vi "Read Cubes.vi"(8 "error in (no error)":errorcluster, 11 "Cubes in":refnum<class "Cubes.lvclass">) -> (0 "error out":errorcluster, 2 "Cubes":refnum<class "Cube.lvclass">[](array[class]), 3 "Cubes out":refnum<class "Cubes.lvclass">)   [LabVIEW 2019, in "22.lvlib" / "Cubes.lvclass"]
uses:
  Cubes.lvclass
  Cube/Cube.lvclass
  Cubes.lvclass/Cubes.ctl
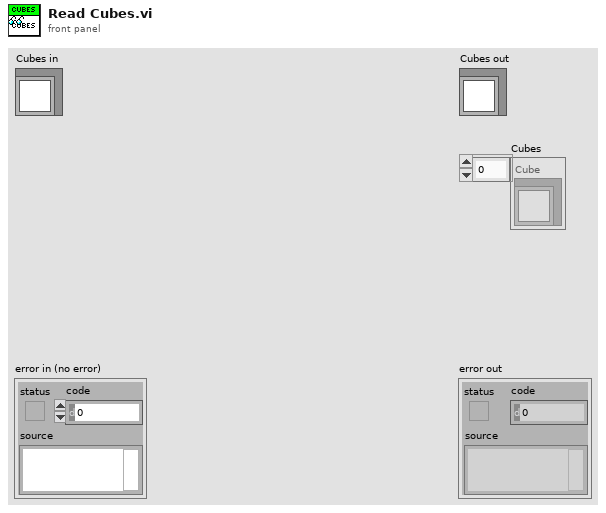
[diagram p1: front panel]
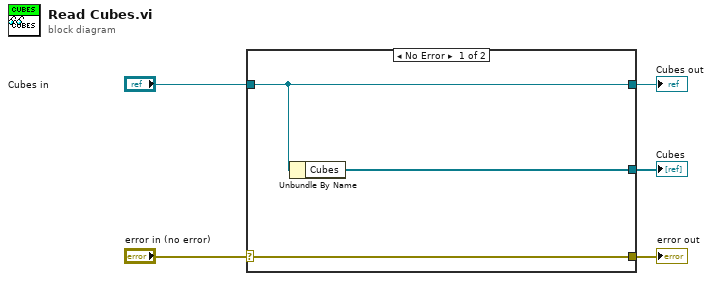
[diagram p0: block diagram]
diagram:
  n1 = case shown="No Error" "error in (no error)" {
    selector: "error in (no error)" -> [w8 w9]
    tunnel: [w8 w9] -> w4
    tunnel: [w7 w10] -> w2
    tunnel: "Cubes in" -> [w7 w10]
    tunnel: [w6 _] -> w1
    frame No Error {
      n2 = Unbundle By Name(w7) -> ("Cubes"=w6:refnum<class "Cube.lvclass">[])
    }
    frame Error {
    }
  }
  "error out" <- w4
  "Cubes out" <- w2
  "Cubes" <- w1
